vi "b-fields many sensors.vi"(0 "magnet location params":T1, 9 "param vector in":dbl[](array[numeric]), 11 "Magnetometer reading set":T2) -> (4 "predicted field":dbl[][](array[numeric]), 6 "pf - flat":dbl[](array[numeric]), 8 "measured field":dbl[][](array[numeric]), 10 "mf - flat":dbl[](array[numeric]), 13 "derivative":dbl[][](array[numeric]), 14 "square error":dbl, 15 "param vector out":dbl[](array[numeric]))   [LabVIEW 2017]
uses:
  typedefs/magnetomter reading set.ctl
  typedefs/magnet location fit result.ctl
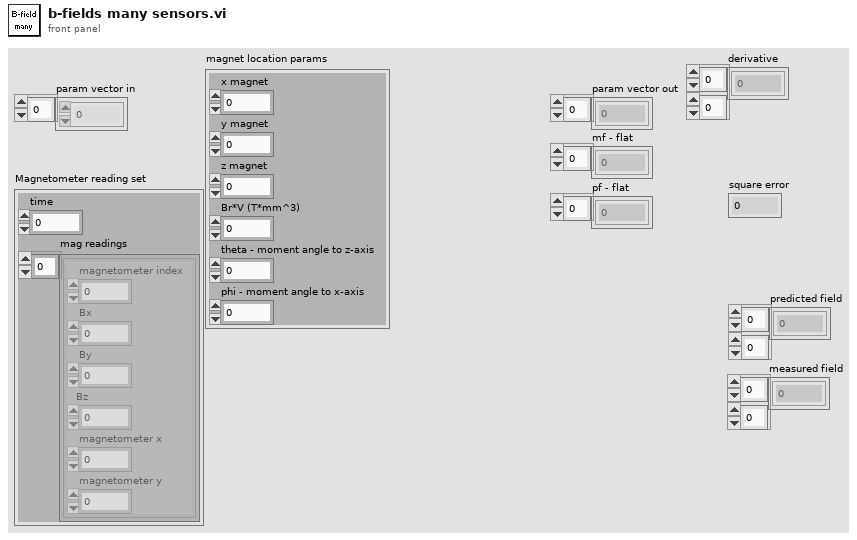
[diagram p1: front panel]
types:
  T1 = typedef "magnet location fit result.ctl" = cluster{"x magnet":dbl, "y magnet":dbl, "z magnet":dbl, "Br*V (T*mm^3)":dbl, "theta - moment angle to z-axis":dbl, "phi - moment angle to x-axis":dbl}
  T2 = typedef "magnetomter reading set.ctl" = cluster{"time":fxp<+,48,48>, "mag readings":cluster{"magnetometer index":dbl, "Bx":dbl, "By":dbl, "Bz":dbl, "magnetometer x":dbl, "magnetometer y":dbl}[]}
  T3 = cluster{"param vector in[0]":dbl, "param vector in[1]":dbl, "param vector in[2]":dbl, "param vector in[3]":dbl, "param vector in[4]":dbl, "param vector in[5]":dbl}
  T4 = cluster{"magnetometer index":dbl, "Bx":dbl, "By":dbl, "Bz":dbl, "magnetometer x":dbl, "magnetometer y":dbl}[]
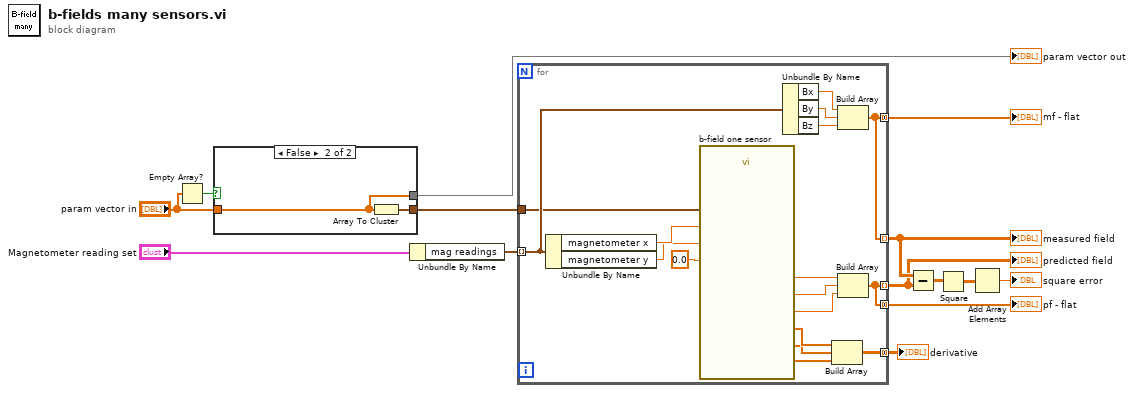
[diagram p0: block diagram]
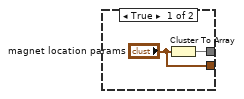
[diagram p2: hidden frame]
diagram:
  n1 = Empty Array?(array="param vector in") -> (empty?=w6:bool)
  n2 = case shown="False" w6 {
    tunnel: [w15 w18] -> w8
    tunnel: "param vector in" -> [_ w18]
    tunnel: ["magnet location params" w17] -> w2
    frame True {
      n3 = Cluster To Array(cluster="magnet location params") -> (array=w15:dbl[])
    }
    frame False {
      n4 = Array To Cluster(array=w18) -> (cluster=w17:T3)
    }
  }
  "param vector out" <- w8
  n5 = Unbundle By Name("Magnetometer reading set") -> ("mag readings"=w14:T4)
  n6 = for {
    tunnel: w14 -> [w32] mode=indexing
    tunnel: [w25] -> w13 mode=indexing
    tunnel: [w24] -> w12 mode=indexing
    tunnel: [w25] -> w4 mode=concatenating
    tunnel: [w24] -> w3 mode=concatenating
    tunnel: w2 -> [w23]
    tunnel: [w19] -> w1 mode=concatenating
    n7 = Unbundle By Name(w32) -> ("magnetometer x"=w35:dbl, "magnetometer y"=w34:dbl)
    n8 = call "b-field one sensor.vi"("magnet location params"=w23, "x sensor"=w35, "y sensor"=w34, "z sensor"=0.0) -> ("Bx (uT)"=w28:dbl, "By (uT)"=w27:dbl, "Bz (uT)"=w26:dbl, "dBx"=w22:dbl[], "dBy"=w21:dbl[], "dBz"=w20:dbl[])  [unwired: 18 in]
    n9 = Unbundle By Name(w32) -> ("Bx"=w31:dbl, "By"=w30:dbl, "Bz"=w29:dbl)
    n10 = Build Array(w22, w21, w20) -> (w19:dbl[][])
    n11 = Build Array(w31, w30, w29) -> (w25:dbl[])
    n12 = Build Array(w28, w27, w26) -> (w24:dbl[])
  }
  "measured field" <- w13
  "predicted field" <- w12
  "mf - flat" <- w4
  "pf - flat" <- w3
  "derivative" <- w1
  n13 = Subtract(x=w13, y=w12) -> (x-y=w11:dbl[][])
  n14 = Square(x=w11) -> (x^2=w10:dbl[][])
  n15 = Add Array Elements(numeric array=w10) -> (sum=→"square error":dbl)
